vi "SystemEinstellungenV2Gasteiler lesen.vi"(8 "Fehler (Eingang)":errorcluster, 9 "Tabellen-String":string, 11 "[GasteilerDefinition]":string) -> (0 "Fehler (Ausgang)":errorcluster, 3 "[GasteilerDefinition]":string[][](array[string]))   [LabVIEW 2020, in "System Einstellungen V2.lvlib"]
uses:
  System Einstellungen V2.lvlib
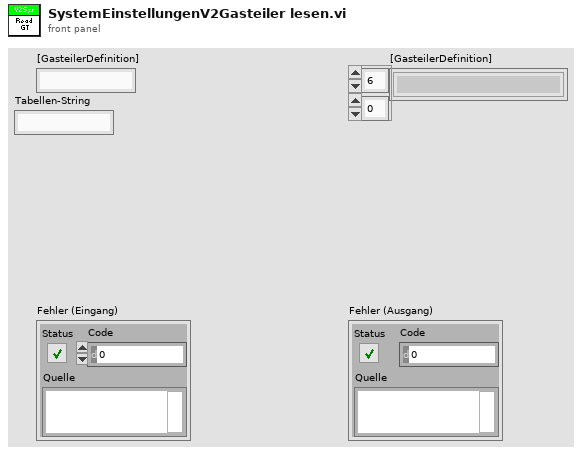
[diagram p1: front panel]
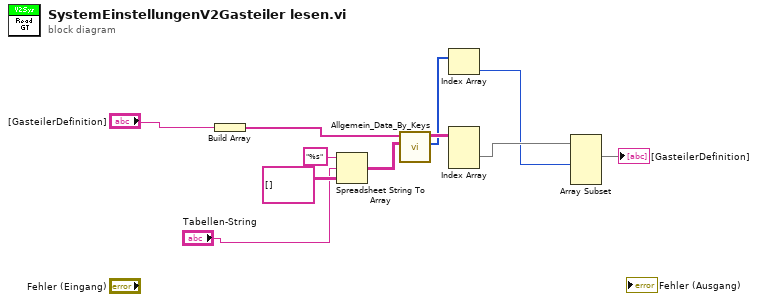
[diagram p0: block diagram]
diagram:
  n1 = Build Array("[GasteilerDefinition]") -> (w8:string[])
  n2 = Spreadsheet String To Array(format string="%s" ("Format-String"), spreadsheet string="Tabellen-String", array type (2D Dbl)=string[][] [] ("String")) -> (array=w11:string[][])  [unwired: 1 in]
  n3 = call "Allgemein_Data_By_Keys.vi"("String"=w11, "Keys (Eingang)"=w8) -> ("Length Array  (Ausgang)"=w3:i32[], "Array (Ausgang)"=w6:string[][][])  [unwired: 8 in]
  n4 = Index Array(array=w3) -> (element=w2:i32)  [unwired: 1 in]
  n5 = Index Array(array=w6) -> (element=w4:string[][])  [unwired: 3 in]
  n6 = Array Subset(array=w4, length (row)=w2) -> (→"[GasteilerDefinition]":string[][])  [unwired: 3 in]
